vi "TestPurePursuit.vi"() -> ()   [LabVIEW 2017]
panel:
  out "Waveform Chart":dbl(graph)
  in  "Gains":T1={"FFV"=0.0088, "FFA"=0.0017, "Vel PID"={"P"=0.02, "I"=0.0, "D"=0.0}} {"Vel PID"."D" format="%.5f"; "Vel PID"."I" format="%.3f"; "Vel PID"."P" format="%.3f"}
  out "Graph":cluster{cluster{"x":dbl, "y":dbl}[]}[](graph)=[{[{"x"=0.0, "y"=0.0}, {"x"=6.000012995757895, "y"=1.8600513921972217e-05}, {"x"=12.000013228274508, "y"=1.8024445399896824e-05}, {"x"=18.000000928025898, "y"=-3.466844065898593e-07}, {"x"=23.999988050149735, "y"=-1.8732899115180867e-05}, {"x"=29.999983497056913, "y"=-2.4626235766886108e-05}, {"x"=35.99998641239224, "y"=-1.9937329750402042e-05}, {"x"=41.999989878071176, "y"=-1.5014976429891381e-05}, {"x"=47.99998780235442, "y"=-1.8516604869522952e-05}, {"x"=53.999978256850234, "y"=-3.2861672539738014e-05}, {"x"=59.999962080988986, "y"=-5.662301937832198e-05}, {"x"=65.99993967758888, "y"=-8.93241306997219e-05}, {"x"=71.99990910478697, "y"=-0.00013409671700333547}, {"x"=77.99986633439214, "y"=-0.00019708755768237262}, {"x"=83.99980649266169, "y"=-0.000285511602173958}, {"x"=89.9997244225526, "y"=-0.00040684498386790204}, {"x"=95.99961375836568, "y"=-0.0005702988579481974}, {"x"=101.99946482837831, "y"=-0.0007900224585265264}, {"x"=107.99926223705762, "y"=-0.0010887187978819172}, {"x"=113.99898272916002, "y"=-0.001500774329040284}, {"x"=119.9985932498305, "y"=-0.0020750587007514485}, {"x"=125.99804847792912, "y"=-0.002878502442261767}, {"x"=131.99728682123086, "y"=-0.004001973825626965}, {"x"=137.99622391478334, "y"=-0.005569875682643498}, {"x"=143.9947428363391, "y"=-0.0077546091500685236}, {"x"=149.99268027923097, "y"=-0.01079700452088169}, {"x"=155.98980762441013, "y"=-0.015034263523333716}, {"x"=161.98580517816765, "y"=-0.020937963202312008}, {"x"=167.98022682402237, "y"=-0.029166183273550337}, {"x"=173.97245101398596, "y"=-0.04063577659197116}, {"x"=179.96161236266764, "y"=-0.056623254058974636}, {"x"=185.94650595963486, "y"=-0.07890592025282842}, {"x"=191.9254536101153, "y"=-0.10995917657701425}, {"x"=197.89611710769913, "y"=-0.1532319618353457}, {"x"=203.85523823484542, "y"=-0.21353027437700015}, {"x"=209.79827504330788, "y"=-0.2975536867575931}, {"x"=215.71890145282623, "y"=-0.4146334560908717}, {"x"=221.6082918041485, "y"=-0.5777878647143637}, {"x"=227.4541653744127, "y"=-0.8051315515384897}, {"x"=233.23938633098282, "y"=-1.1219407087112445}, {"x"=238.9400934087892, "y"=-1.5634118263787973}, {"x"=244.52303497248954, "y"=-2.17859262350257}, {"x"=249.94186710076684, "y"=-3.0358425771324073}, {"x"=255.13201459168647, "y"=-4.230413080366287}, {"x"=260.0034978546561, "y"=-5.895028438265746}, {"x"=264.43092635445544, "y"=-8.214645080668248}, {"x"=268.239571852254, "y"=-11.446996245449666}, {"x"=271.60501644884937, "y"=-15.332256752193304}, {"x"=274.6536121006905, "y"=-19.683127514985774}, {"x"=277.47649545692303, "y"=-24.364057716740298}, {"x"=280.1397247827417, "y"=-29.27616828010769}, {"x"=282.6916222274472, "y"=-34.34626266034073}, {"x"=285.16813701665603, "y"=-39.518702153385135}, {"x"=287.5968418343859, "y"=-44.74922040942905}, {"x"=290.0, "y"=-50.0}]}, {[{"x"=291.1533460219868, "y"=-53.33257445451973}, {"x"=295.95554084093766, "y"=-64.32979796415349}]}, {[{"x"=290.0, "y"=-50.0}]}, {[{"x"=306.1533460219868, "y"=-53.33257445451973}, {"x"=305.4191937664141, "y"=-48.69731953889552}, {"x"=303.288600937611, "y"=-44.51579567013263}, {"x"=299.9701248063739, "y"=-41.19731953889551}, {"x"=295.788600937611, "y"=-39.066726710092425}, {"x"=291.1533460219868, "y"=-38.33257445451973}, {"x"=286.5180911063626, "y"=-39.066726710092425}, {"x"=282.3365672375997, "y"=-41.19731953889551}, {"x"=279.0180911063626, "y"=-44.51579567013263}, {"x"=276.88749827755953, "y"=-48.69731953889551}, {"x"=276.1533460219868, "y"=-53.33257445451973}, {"x"=276.88749827755953, "y"=-57.96782937014394}, {"x"=279.0180911063626, "y"=-62.149353238906826}, {"x"=282.3365672375997, "y"=-65.46782937014395}, {"x"=286.5180911063626, "y"=-67.59842219894703}, {"x"=291.1533460219868, "y"=-68.33257445451973}, {"x"=295.788600937611, "y"=-67.59842219894703}, {"x"=299.9701248063739, "y"=-65.46782937014395}, {"x"=303.288600937611, "y"=-62.149353238906826}, {"x"=305.4191937664141, "y"=-57.967829370143946}, {"x"=306.1533460219868, "y"=-53.33257445451974}]}, {[{"x"=257.1744147922948, "y"=109.38907794991484}, {"x"=277.07572619628826, "y"=-16.26285707106871}, {"x"=334.83158138745586, "y"=-129.61510522368843}, {"x"=424.7884348509808, "y"=-219.57195868721334}, {"x"=538.1406830036004, "y"=-277.32781387838094}, {"x"=663.792618024584, "y"=-297.2291252823744}, {"x"=789.4445530455675, "y"=-277.32781387838094}, {"x"=902.7968011981873, "y"=-219.57195868721334}, {"x"=992.7536546617122, "y"=-129.6151052236885}, {"x"=1050.5095098528798, "y"=-16.26285707106875}, {"x"=1070.4108212568733, "y"=109.38907794991478}, {"x"=1050.5095098528798, "y"=235.04101297089835}, {"x"=992.7536546617123, "y"=348.3932611235181}, {"x"=902.7968011981874, "y"=438.350114587043}, {"x"=789.4445530455677, "y"=496.10596977821064}, {"x"=663.7926180245842, "y"=516.0072811822041}, {"x"=538.1406830036005, "y"=496.10596977821064}, {"x"=424.7884348509809, "y"=438.3501145870431}, {"x"=334.8315813874559, "y"=348.3932611235182}, {"x"=277.07572619628826, "y"=235.04101297089846}, {"x"=257.1744147922948, "y"=109.38907794991493}]}]
  in  "Max Accel":dbl=120.0 format="%#_13g"
  in  "MaxVel":dbl(slide)=120.0 scale=0.0..100.0
  in  "LookAhead":dbl=15.0
  in  "Path":cluster{"x":dbl, "y":dbl}[](array[cluster])=[{"x"=0.0, "y"=0.0}, {"x"=270.0, "y"=0.0}, {"x"=290.0, "y"=-50.0}]
  in  "Config":T2={"Gear Reduction"=15.0, "Wheel Radius (m)"=0.076, "# Motors"=1, "coeff of friction"=0.1, "Mass (kg)"=50.0, "Motor"={"Ke (V)"=0.0183, "R (ohms)"=0.09, "KT (Nm/A)"=0.0183, "Tf (Nm)"=0.4}}
  # ".007"
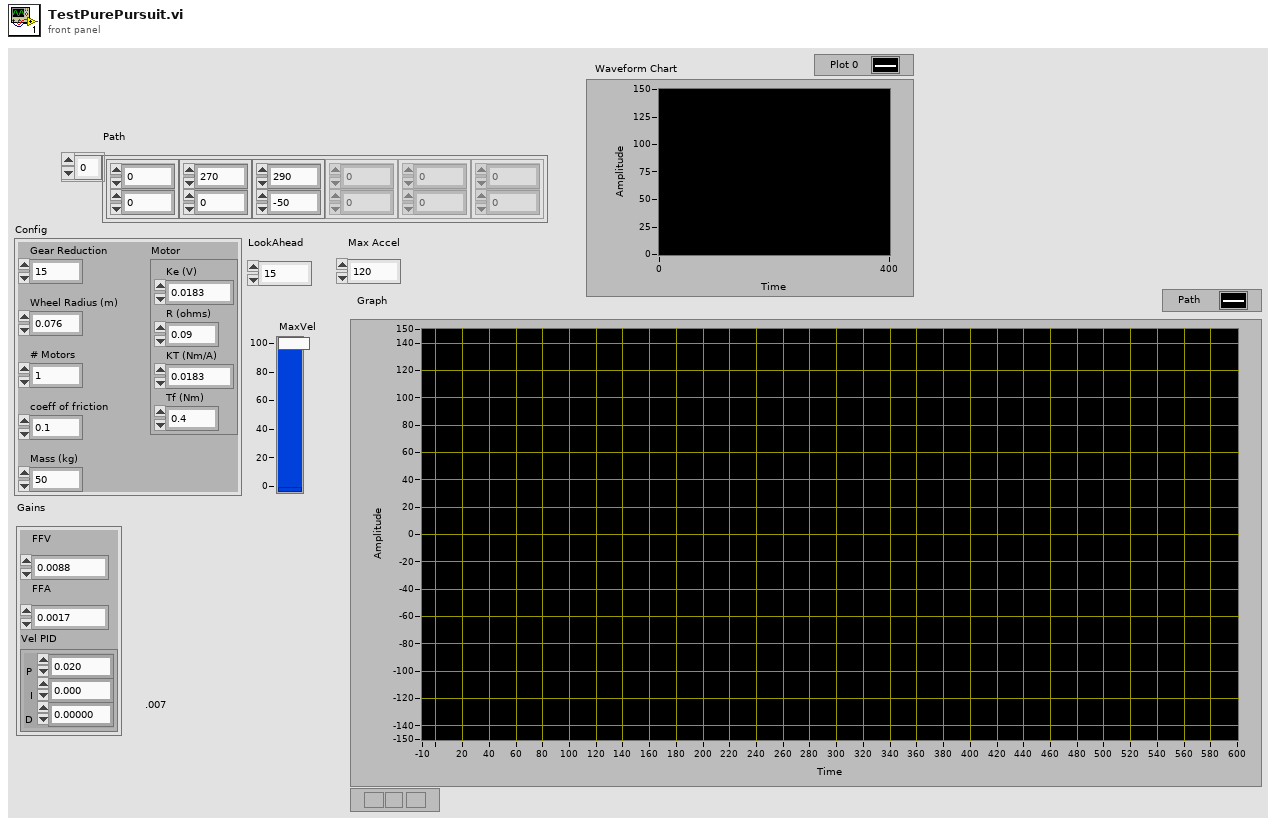
[diagram p1: front panel]
types:
  T1 = cluster{"FFV":dbl, "FFA":dbl, "Vel PID":cluster{"P":dbl, "I":dbl, "D":dbl}}
  T2 = cluster{"Gear Reduction":dbl, "Wheel Radius (m)":dbl, "# Motors":u32, "coeff of friction":dbl, "Mass (kg)":dbl, "Motor":cluster{"Ke (V)":dbl, "R (ohms)":dbl, "KT (Nm/A)":dbl, "Tf (Nm)":dbl}}
  T3 = cluster{"SmoothPath":cluster{dbl, dbl}[], "Distance":dbl, "DistancesToEnd":dbl[], "Vel":dbl[]}
  T4 = cluster{"LeftDistance":dbl, "RightDistance":dbl, "LeftVelocity":dbl, "RightVelocity":dbl, "Angle":dbl, "Location":cluster{dbl, dbl}}
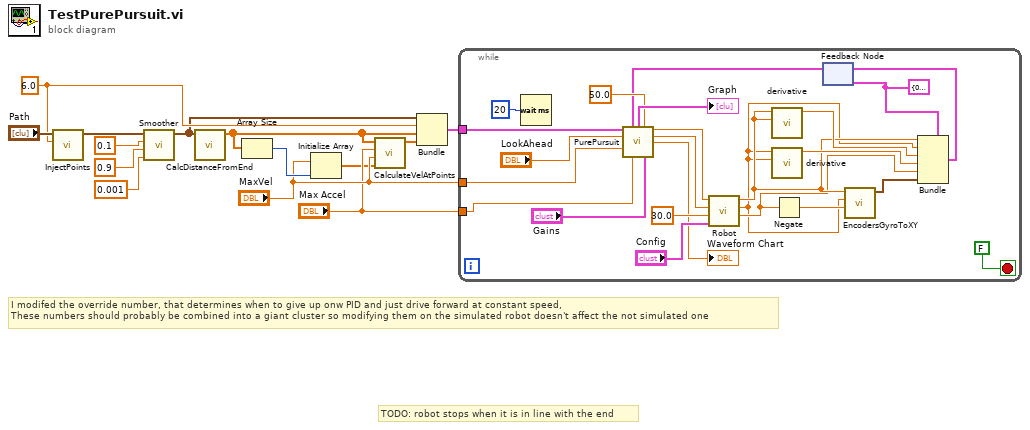
[diagram p0: block diagram]
diagram:
  w10 = 6.0 ("Distance")
  # "TODO: robot stops when it is in line with the end"
  # "I modifed the override number, that determines when to give up onw PID and just drive forward at constant speed,\nThese numbers should probably be combined into a giant cluster so modifying them on the simulated robot doesn't affect the not simulated one"
  n1 = call "InjectPoints.vi"("Spacing"=w10, "Path"="Path") -> ("Path out"=w8:cluster{dbl, dbl}[])  [unwired: 9 in]
  n2 = call "Smoother.vi"("tolerance"=0.001, "B"=0.9, "A"=0.1, "Path"=w8) -> ("SmoothPath"=w7:cluster{dbl, dbl}[])  [unwired: 7 in]
  n3 = call "CalcDistanceFromEnd.vi"("Path"=w7) -> ("DistancesToEnd"=w6:dbl[])  [unwired: 10 in]
  n4 = Array Size(array=w6) -> (size(s)=w5:i32)
  n5 = Initialize Array("MaxVel", w5) -> (w1:dbl[])
  n6 = call "CalculateVelAtPoints.vi"("MaxVels"=w1, "MaxVel"="MaxVel", "MaxAccel"="Max Accel", "DistancesToEnd"=w6) -> ("Vel"=w2:dbl[])  [unwired: 7 in]
  n7 = Bundle("SmoothPath"=w7, "Distance"=w10, "DistancesToEnd"=w6, "Vel"=w2) -> (w9:T3)  [unwired: 1 in]
  n8 = while {
    tunnel: w9 -> [w36]
    tunnel: "MaxVel" -> [w27]
    tunnel: "Max Accel" -> [w26]
    stop <- FALSE stop-if-true
    w23 = T4 {"LeftDistance"=0.0, "RightDistance"=0.0, "LeftVelocity"=0.0, "RightVelocity"=0.0, "Angle"=0.0, "Location"={0.0, 0.0}} ("SensorData")
    n9 = Wait (ms)(milliseconds to wait=u32 20) -> ()  [unwired: 1 out]
    n10 = feedback #1(w23) -> (w17:T4)
    n11 = call "PurePursuit.vi"("PathData"=w36, "SensorData"=w17, "Trackwidth"=50.0, "LookAhead"="LookAhead", "MaxVel"=w27, "Max Accel"=w26, "Gains"="Gains") -> ("Graph"=→"Graph":cluster{cluster{"x":dbl, "y":dbl}[]}[], "LeftValue"=w34:dbl, "RightValue"=w33:dbl, "TargetVel"=→"Waveform Chart":dbl)  [unwired: 3 in, 2 out]
    n12 = call "Robot.vi"("Config"="Config", "WheelBase"=30.0, "Right Value"=w33, "Left Value"=w34) -> ("Angle"=w16:dbl, "Right Distance"=w15:dbl, "Left Distance"=w20:dbl)  [unwired: 5 in]
    n13 = call "derivative.vi"("Starting value"=w20, "x"=w20) -> ("dx/dt"=w22:dbl)  [unwired: 9 in]
    n14 = call "derivative.vi"("Starting value"=w15, "x"=w15) -> ("dx/dt"=w21:dbl)  [unwired: 9 in]
    n15 = Negate(x=w16) -> (-x=w19:dbl)
    n16 = call "EncodersGyroToXY.vi"("Angle (degrees)"=w19, "Right Distance"=w15, "Left Distance"=w20) -> ("Location"=w18:cluster{dbl, dbl})  [unwired: 7 in, 1 out]
    n17 = Bundle(cluster=w23, "LeftDistance"=w20, "RightDistance"=w15, "LeftVelocity"=w22, "RightVelocity"=w21, "Angle"=w16, "Location"=w18) -> (w31:T4)
    n18 = feedback-in #1(w31) -> ()
  }
